vi "Cure.vi"(6 "Variant in":variant, 7 "Shift Pressed?":bool, 8 "error in (no error)":errorcluster, 10 "QD Combo Box Ref":refnum<vi>, 11 "QD Launch VI Ref":refnum<vi>) -> (0 "error out":errorcluster, 4 "Variant out":variant)   [LabVIEW 2017, in "Quick Drop.lvlib"]
doc: "Cures the grave site (Diagram Disable structure) of the zombie (enabled legacy code) infection. The Spirit frame (refactored code) is enabled and the Zombie frame is disabled. No timestamps or labels are changed. This is the opposite of infecting a grave site with a zombie virus.\n\nDefault Shortcut - [C]"
uses:
  Quick Drop.lvlib
  Eulogy/Eulogy.lvlib
panel:
  in  "Undo Name":string="Cure"
  # "Do not change the connector pane of this VI.\n\nSee the block diagram for directions on how to use this template."
  # "Specify the name of the Undo transaction"
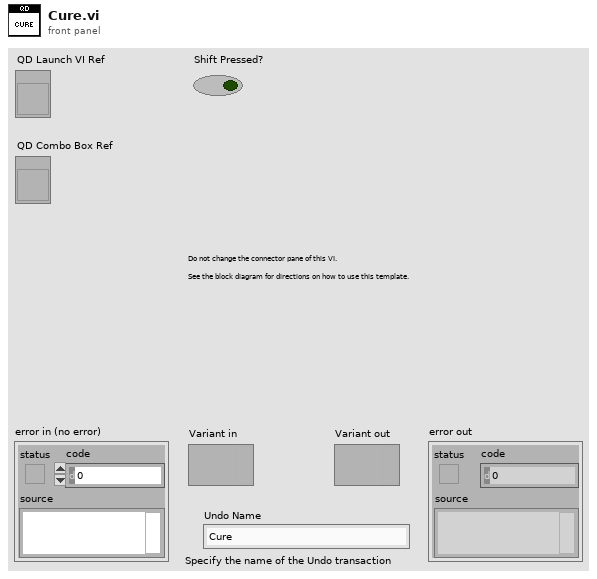
[diagram p1: front panel]
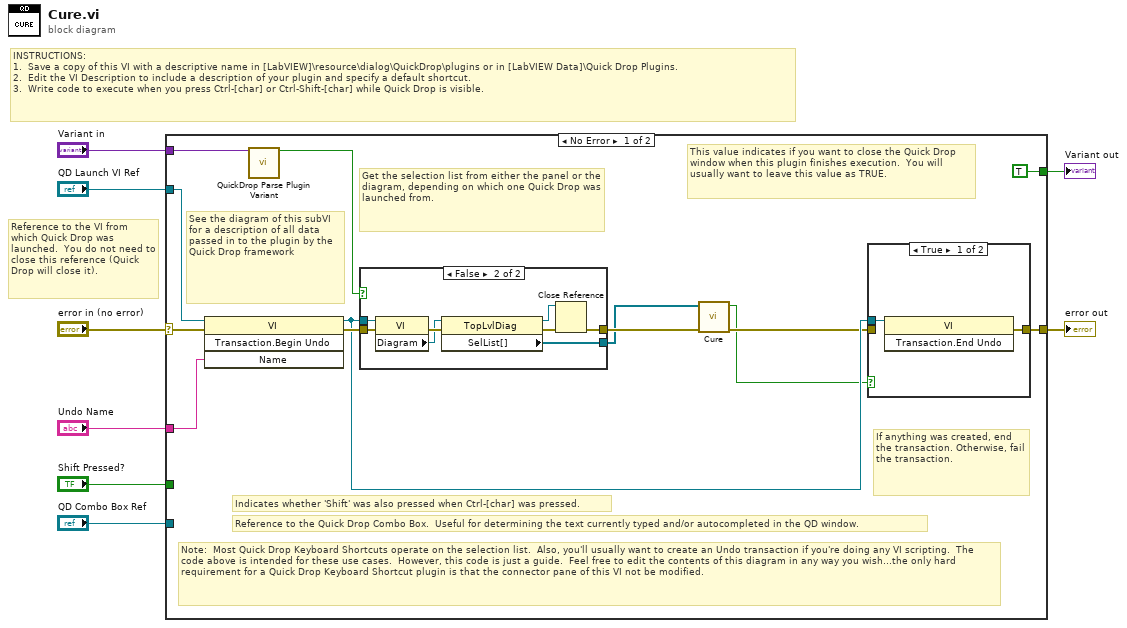
[diagram p0: block diagram]
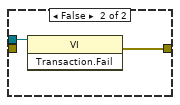
[diagram p2: hidden frame]
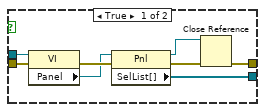
[diagram p3: hidden frame]
diagram:
  # "Reference to the VI from which Quick Drop was launched.  You do not need to close this reference (Quick Drop will close it)."
  # "INSTRUCTIONS:\n1.  Save a copy of this VI with a descriptive name in [LabVIEW]\\resource\\dialog\\QuickDrop\\plugins or in [LabVIEW Data]\\Quick Drop Plugins.\n2.  Edit the VI Description to include a description of your plugin and specify a default shortcut. \n3.  Write code to execute when you press Ctrl-[char] or Ctrl-Shift-[char] while Quick Drop is visible."
  n1 = case shown="No Error" "error in (no error)" {
    selector: "error in (no error)" -> [w20 w42]
    tunnel: [w14 w42] -> w7
    tunnel: "QD Launch VI Ref" -> [w19 _]
    tunnel: "Shift Pressed?" -> [_ _]
    tunnel: "QD Combo Box Ref" -> [_ _]
    tunnel: "Variant in" -> [w21 _]
    tunnel: "Undo Name" -> [w18 _]
    tunnel: [TRUE _] -> w1
    frame No Error {
      # "Note:  Most Quick Drop Keyboard Shortcuts operate on the selection list.  Also, you'll usually want to create an Undo transaction if you're doing any VI scripting.  The code above is intended for these use cases.  However, this code is just a guide.  Feel free to edit the contents of this diagram in any way you wish...the only hard requirement for a Quick Drop Keyboard Shortcut plugin is that the connector pane of this VI not be modified."
      # "Get the selection list from either the panel or the diagram, depending on which one Quick Drop was launched from."
      # "If anything was created, end the transaction. Otherwise, fail the transaction."
      # "This value indicates if you want to close the Quick Drop window when this plugin finishes execution.  You will usually want to leave this value as TRUE."
      # "See the diagram of this subVI for a description of all data passed in to the plugin by the Quick Drop framework"
      # "Reference to the Quick Drop Combo Box.  Useful for determining the text currently typed and/or autocompleted in the QD window."
      # "Indicates whether 'Shift' was also pressed when Ctrl-[char] was pressed."
      n2 = invoke class="VI" method="Transaction.Begin Undo"(reference=w19, error in=w20, "Name"=w18) -> (reference out=w13:refnum<vi>, error out=w15:errorcluster)  [unwired: 1 in, 2 out]
      n3 = call <vilib>:"QuickDrop Parse Plugin Variant.vi"("QDKS Variant in"=w21) -> ("QD Launch VI Panel?"=w16:bool)  [unwired: 12 in, 2 out]
      n4 = case shown="False" w16 {
        tunnel: w15 -> [w33 w41]
        tunnel: w13 -> [w32 w40]
        tunnel: [w27 w35] -> w12
        tunnel: [w26 w34] -> w9
        frame True {
          n5 = property class="VI"(reference=w32, error in=w33) -> (error out=w31:errorcluster, "Panel"=w30:refnum<vi>)  [unwired: 1 out]
          n6 = property class="Pnl"(reference=w30, error in=w31) -> (reference out=w28:refnum<vi>, error out=w29:errorcluster, "SelList[]"=w26:refnum<vi>[])
          n7 = Close Reference(reference=w28, error in (no error)=w29) -> (error out=w27:errorcluster)
        }
        frame False {
          n8 = property class="VI"(reference=w40, error in=w41) -> (error out=w39:errorcluster, "Diagram"=w38:refnum<vi>)  [unwired: 1 out]
          n9 = property class="TopLvlDiag"(reference=w38, error in=w39) -> (reference out=w36:refnum<vi>, error out=w37:errorcluster, "SelList[]"=w34:refnum<vi>[])
          n10 = Close Reference(reference=w36, error in (no error)=w37) -> (error out=w35:errorcluster)
        }
      }
      n11 = call "Cure.vi"("Error In"=w12, "Selection List[]"=w9) -> ("Error Out"=w11:errorcluster, "Change Made?"=w10:bool)  [unwired: 8 in]
      n12 = case shown="True" w10 {
        tunnel: w13 -> [w22 w24]
        tunnel: [w23 w25] -> w14
        tunnel: w11 -> [_ _]
        frame True {
          n13 = invoke class="VI" method="Transaction.End Undo"(reference=w22) -> (error out=w23:errorcluster)  [unwired: 2 in, 2 out]
        }
        frame False {
          n14 = invoke class="VI" method="Transaction.Fail"(reference=w24) -> (error out=w25:errorcluster)  [unwired: 2 in, 2 out]
        }
      }
    }
    frame Error {
    }
  }
  "error out" <- w7
  "Variant out" <- w1
